vi "DB Tools Check If Tbl Exists.vi"(4 "error in (no error)":errorcluster, 6 "table name":string, 7 "connection reference":T1) -> (0 "error out":errorcluster, 2 "exists?":bool, 3 "connection reference out":T1)   [LabVIEW 2017, in "NI_Database_API.lvlib"]
doc: "Checks if a specified table exists in the database specified by the connection reference."
uses:
  <vilib>/addons/database/NI_Database_API.lvlib
  <vilib>/addons/database/Connection.llb/Conn ObjectReference.ctl
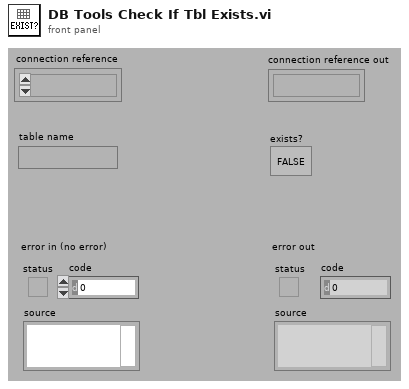
[diagram p1: front panel]
types:
  T1 = typedef "NI_Database_API.lvlib/Conn ObjectReference.ctl" = refnum<k1>
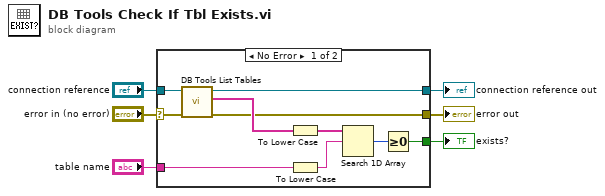
[diagram p0: block diagram]
diagram:
  n1 = case shown="No Error" "error in (no error)" {
    selector: "error in (no error)" -> [w7 w18]
    tunnel: [w15 _] -> w6
    tunnel: "table name" -> [w13 _]
    tunnel: "connection reference" -> [w11 w17]
    tunnel: [w9 w17] -> w3
    tunnel: [w8 w18] -> w2
    frame No Error {
      n2 = call <vilib>:"DB Tools List Tables.vi"("error in (no error)"=w7, "connection reference"=w11) -> ("error out"=w8:errorcluster, "tables"=w10:string[], "connection reference out"=w9:T1)  [unwired: 3 in]
      n3 = To Lower Case(string=w10) -> (all lower case string=w14:string[])
      n4 = To Lower Case(string=w13) -> (all lower case string=w12:string)
      n5 = Search 1D Array(1D array=w14, element=w12) -> (index of element=w16:i32)  [unwired: 1 in]
      n6 = Greater Or Equal To 0?(x=w16) -> (x >= 0?=w15:bool)
    }
    frame Error {
    }
  }
  "connection reference out" <- w3
  "error out" <- w2
  "exists?" <- w6
